vi "PMT_plus_Kiethley.vi"() -> ()   [LabVIEW 2024]
uses:
  <vilib>/Analysis/NI_AALBase.lvlib
  <vilib>/Analysis/1siggen.llb/Ramp Pattern by Delta.vi
  <vilib>/Utility/file.llb/Write Delimited Spreadsheet (string).vi
  <vilib>/Utility/file.llb/Write Delimited Spreadsheet (DBL).vi
  <userlib>/H11890api/H11890api.lvlib
panel:
  in  "Time to wait before current meas (ms)":i32
  in  "Use PMT?":bool=TRUE
  out "XY Graph":cluster{dbl[], dbl[]}(graph)
  out "Actual Voltage":dbl
  in  "Num Current Meas":i32=6
  in  "Path":path
  out "error out":errorcluster
  in  "VISA resource name":refnum<visa-resource-name>
  out "Set Voltage":dbl
  in  "Step Size (V)":dbl=0.1 format="%#_13g"
  in  "Max V":dbl format="%#_13g"
  in  "Start V":dbl format="%#_13g"
  out "current":dbl
  in  "measurement interval":i32=200
  in  "Source Limit Level (0.1)":dbl=5e-08
  out "standard deviation":dbl
  out "mean":dbl
  out "data":u32[](array[numeric])
  out "OLD":bool
  out "DB":u32[](array[numeric])
  out "Overload":i32
  out "Gate Number":i32
  in  "Correction":bool=TRUE
  out "Num Gates Read":i32
  out "Gate Time Read":i32 caption="Gate time Read"
  out "Num Gates Set":i32=20
  out "Gate Time Set":i32=200
  out "PowerD":i32 caption="Power\nRead Data"
  out "Handle Number":i32
  # "as of now it only records every 1V"
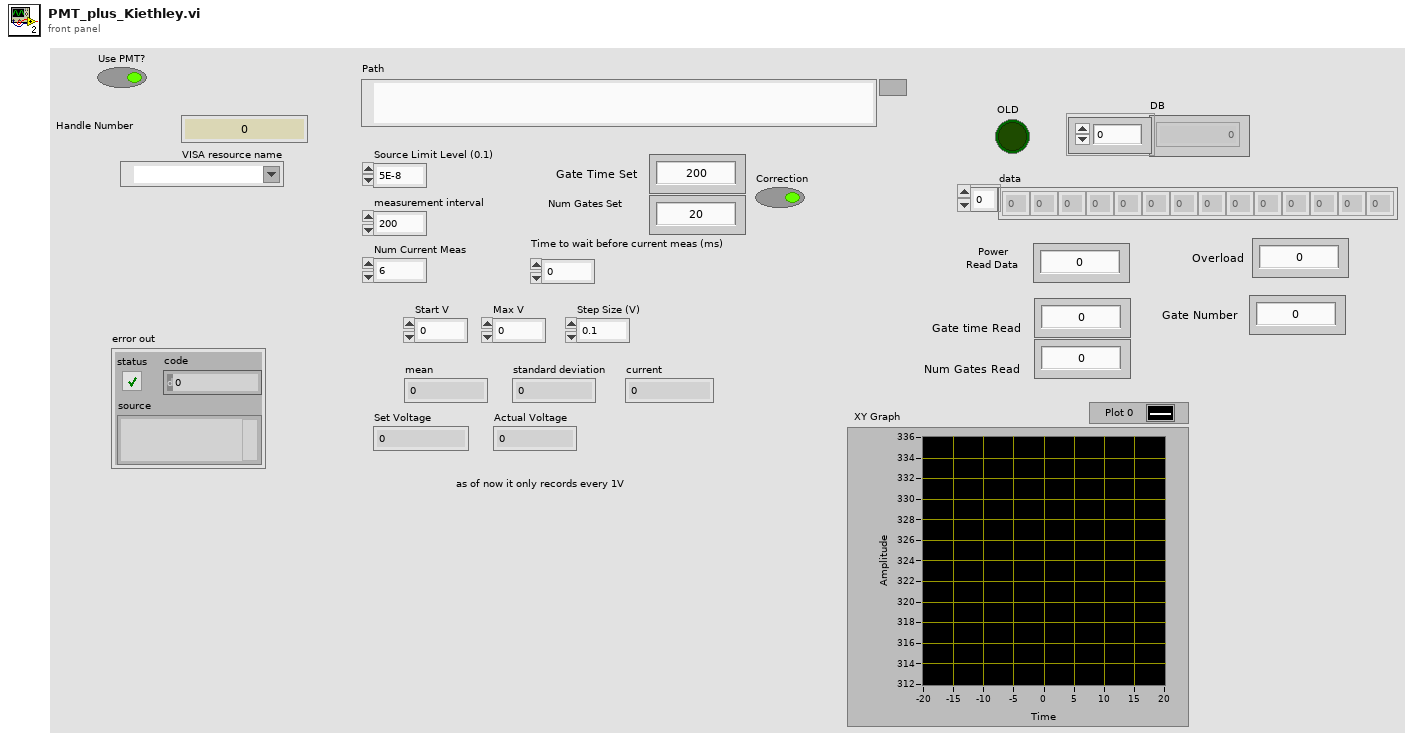
[diagram p1: front panel]
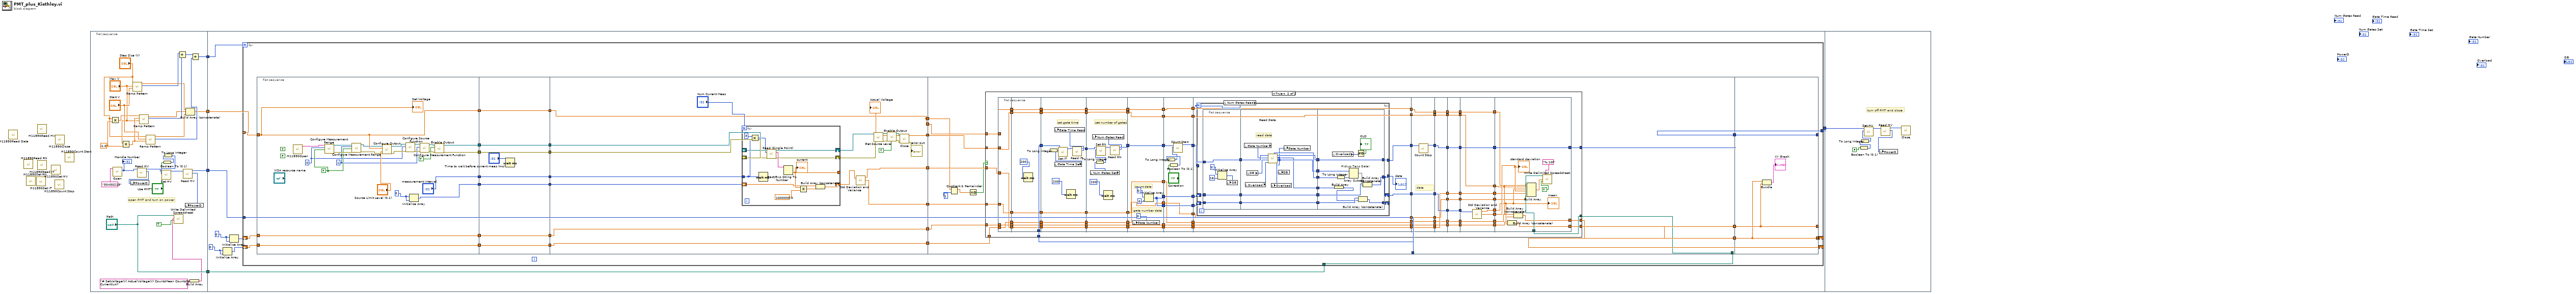
[diagram p0: block diagram]
diagram:
  n1 = call <userlib>:"H11890Read Data.vi"() -> ()  [unwired: 7 in, 5 out]
  n2 = call <userlib>:"H11890Read RN.vi"() -> ()  [unwired: 9 in, 3 out]
  n3 = call <userlib>:"H11890Set RN.vi"() -> ()  [unwired: 10 in, 2 out]
  n4 = call <userlib>:"H11890Set IT.vi"() -> ()  [unwired: 10 in, 2 out]
  n5 = call <userlib>:"H11890Read HV.vi"() -> ()  [unwired: 9 in, 3 out]
  n6 = call <userlib>:"H11890Read IT.vi"() -> ()  [unwired: 9 in, 3 out]
  n7 = call <userlib>:"H11890Set HV.vi"() -> ()  [unwired: 10 in, 2 out]
  n8 = call <userlib>:"H11890Count Stop.vi"() -> ()  [unwired: 10 in, 2 out]
  n9 = call <userlib>:"H11890Close.vi"() -> ()  [unwired: 10 in, 2 out]
  n10 = call <userlib>:"H11890Count Start.vi"() -> ()  [unwired: 10 in, 2 out]
  n11 = flat-sequence {
    tunnel: [w25] -> w5
    tunnel: [w14] -> w4
    tunnel: [w13] -> w3
    tunnel: ["Path"] -> w1
    tunnel: w5 -> [w43]
    tunnel: w4 -> [w42]
    tunnel: w3 -> [w41]
    tunnel: [w40] -> w2
    tunnel: w1 -> [w39]
    tunnel: w2 -> [w434]
    frame #0 {
      w8 = -1.0
      # "open PMT and turn on power"
      n12 = Multiply(x="Step Size (V)", y=w8) -> (x*y=w6:dbl)
      n13 = call "Open.vi"("Serial Number"="30430219") -> ("Handle Number"=w29:i32)  [unwired: 9 in, 1 out]
      "Handle Number" <- w29
      n14 = Multiply(x="Max V", y=w8) -> (x*y=w16:dbl)
      n15 = call-poly <vilib>:"Ramp Pattern.vi"("start"="Start V", "end"="Max V", "delta"="Step Size (V)") -> ("samples"=w21:i32, "Ramp Pattern"=w18:dbl[])  [unwired: 6 in, 1 out]
      n16 = call "Read HV.vi"("handle"=w29) -> ("HV out"=w28:i32, "handle out"=w32:i32)  [unwired: 8 in, 1 out]
      n17 = local write "PowerD"(w28) -> ()
      n18 = call-poly <vilib>:"Ramp Pattern.vi"("start"="Max V", "end"=w16, "delta"=w6) -> ("samples"=w22:i32, "Ramp Pattern"=w19:dbl[])  [unwired: 6 in, 1 out]
      n19 = call-poly <vilib>:"Ramp Pattern.vi"("start"=w16, "end"="Start V", "delta"="Step Size (V)") -> ("samples"=w24:i32, "Ramp Pattern"=w20:dbl[])  [unwired: 6 in, 1 out]
      n20 = Boolean To (0,1)(Boolean="Use PMT?") -> (0, 1=w30:i16)
      n21 = To Long Integer(number=w30) -> (32bit integer=w31:i32)
      n22 = call "Set HV.vi"("HV"=w31, "handle"=w32) -> ("handle out"=w34:i32)  [unwired: 8 in, 1 out]
      n23 = Add(x=w21, y=w22) -> (x+y=w23:i32)
      n24 = call "Read HV.vi"("handle"=w34) -> ("HV out"=w33:i32, "handle out"=w25:i32)  [unwired: 8 in, 1 out]
      n25 = local write "PowerD"(w33) -> ()
      n26 = Build Array (concatenate)(w18, w19, w20) -> (w14:dbl[])
      n27 = Build Array("# SetVoltage(V) ActualVoltage(V) CountsMean CountsStd Current(uA)") -> (w10:string[])
      n28 = call-poly <vilib>:"Write Delimited Spreadsheet.vi"("file path (dialog if empty)"="Path", "1D data"=w10, "append to file? (new file:F)"=TRUE) -> ()  [unwired: 11 in, 2 out]
      n29 = Add(x=w23, y=w24) -> (x+y=w13:i32)
    }
    frame #1 {
      w37 = 0
      w38 = 0
      n30 = Initialize Array(w37, w37) -> (w36:i32[])
      n31 = Initialize Array(w38, w38) -> (w35:i32[])
      n32 = for {
        N: w41 -> [_]
        tunnel: w42 -> [w75] mode=indexing
        tunnel: w43 -> [w74]
        tunnel: [w73] -> w40
        tunnel: w39 -> [w72]
        shift-right: [w59] -> _
        shift-left: w35 -> [w67]
        shift-right: [w60] -> _
        shift-left: w36 -> [w66]
        n33 = flat-sequence {
          tunnel: w66 -> [w99]
          tunnel: w67 -> [w100]
          tunnel: w75 -> [w101]
          tunnel: [w101] -> w58
          tunnel: [w100] -> w56
          tunnel: [w99] -> w54
          tunnel: ["measurement interval"] -> w52
          tunnel: [w79] -> w50
          tunnel: [w78] -> w48
          tunnel: [w77] -> w46
          tunnel: w58 -> [w109]
          tunnel: [w109] -> w57
          tunnel: w56 -> [w108]
          tunnel: [w108] -> w55
          tunnel: w54 -> [w107]
          tunnel: [w107] -> w53
          tunnel: w52 -> [w106]
          tunnel: [w106] -> w51
          tunnel: w50 -> [w105]
          tunnel: [w105] -> w49
          tunnel: w48 -> [w104]
          tunnel: [w104] -> w47
          tunnel: w46 -> [w103]
          tunnel: [w103] -> w45
          tunnel: [w119] -> w71
          tunnel: [w120] -> w70
          tunnel: [w112] -> w69
          tunnel: [w119] -> w68
          tunnel: [w118] -> w65
          tunnel: [w117] -> w64
          tunnel: w57 -> [w119]
          tunnel: w55 -> [w118]
          tunnel: w53 -> [w117]
          tunnel: w51 -> [w116]
          tunnel: w49 -> [w115]
          tunnel: w47 -> [w114]
          tunnel: w45 -> [w113]
          tunnel: [w110] -> w44
          tunnel: w74 -> [w157]
          tunnel: w72 -> [w155]
          tunnel: w71 -> [w154]
          tunnel: w70 -> [w153]
          tunnel: w69 -> [w152]
          tunnel: w68 -> [w149]
          tunnel: w65 -> [w147]
          tunnel: w64 -> [w146]
          tunnel: [w156] -> w63
          tunnel: [w145] -> w62
          tunnel: [w144] -> w61
          tunnel: w44 -> [w143]
          tunnel: [w431] -> w59
          tunnel: [w432] -> w60
          tunnel: [w433] -> w73
          tunnel: w63 -> [w433]
          tunnel: w62 -> [w432]
          tunnel: w61 -> [w431]
          frame #0 {
            w85 = 0
            w84 = TRUE
            w81 = 1
            w83 = 0
            (unwired) FALSE
            (unwired) TRUE
            n34 = call <userlib>:"H11890Open.vi"() -> ("cSerialNumber out"=w76:string)  [unwired: 10 in, 1 out]
            n35 = call "Configure Measurement Range.vi"("Enable Auto Range (T:Enable)"=w84, "Function (0: Volts)"=w83, "VISA resource name"=w76) -> ("error out"=w96:errorcluster, "VISA resource name out"=w95:refnum<visa-resource-name>, "error in (no error)"=w97:errorcluster)  [unwired: 6 in]
            n36 = call "Configure Measurement Range.vi"("error in (no error)"=w96, "Enable Auto Range (T:Enable)"=w84, "Function (0: Volts)"=w81, "VISA resource name"=w95) -> ("error out"=w91:errorcluster, "VISA resource name out"=w87:refnum<visa-resource-name>)  [unwired: 6 in]
            n37 = call "Configure Output.vi"("VISA resource name"=w87, "Source Level (0)"=w101, "Source Limit Level (0.1)"="Source Limit Level (0.1)", "error in (no error)"=w91) -> ("VISA resource name out"=w88:refnum<visa-resource-name>, "error out"=w92:errorcluster)  [unwired: 10 in]
            n38 = call "Configure Source Function.vi"("error in (no error)"=w92, "Function (0: Volts)"=w83, "VISA resource name"=w88) -> ("error out"=w93:errorcluster, "VISA resource name out"=w89:refnum<visa-resource-name>)  [unwired: 7 in]
            n39 = Initialize Array(w85, w85) -> (w79:i32[])
            n40 = call "Configure Measurement Function.vi"("error in (no error)"=w93, "Function (0: Volts)"=w81, "VISA resource name"=w89) -> ("error out"=w94:errorcluster, "VISA resource name out"=w90:refnum<visa-resource-name>)  [unwired: 7 in]
            n41 = call "Enable Output.vi"("error in (no error)"=w94, "Enable Output (T: Enable)"=TRUE, "VISA resource name"=w90) -> ("error out"=w78:errorcluster, "VISA resource name out"=w77:refnum<visa-resource-name>)  [unwired: 7 in]
            "Set Voltage" <- w101
          }
          frame #1 {
            n42 = Wait (ms)(milliseconds to wait="Time to wait before current meas (ms)") -> ()  [unwired: 1 out]
          }
          frame #2 {
            n43 = for {
              N: "Num Current Meas" -> [_]
              tunnel: [w131] -> _
              shift-right: [w141] -> w126
              shift-left: w114 -> [w140]
              shift-right: [w139] -> w129
              shift-left: w113 -> [w138]
              tunnel: w116 -> [w135]
              shift-right: [w133] -> w111
              shift-left: w115 -> [w134]
              n44 = Multiply(x=3, y=w135) -> (x*y=w137:i32)
              n45 = Wait (ms)(milliseconds to wait=w135) -> ()  [unwired: 1 out]
              n46 = call "Read (Single Point).vi"("VISA resource name"=w138, "Timeout (10000 ms)"=w137, "error in (no error)"=w140) -> ("VISA resource name out"=w139:refnum<visa-resource-name>, "Data out"=w142:string, "error out"=w141:errorcluster)  [unwired: 10 in]
              n47 = Fract/Exp String To Number(string=w142) -> (number=w131:dbl)  [unwired: 3 in, 1 out]
              "current" <- w131
              n48 = Multiply(x=w131, y=1000000.0) -> (x*y=w130:dbl)
              n49 = Build Array (concatenate)(w134, w130) -> (w133:dbl[])
            }
            n50 = call <vilib>:"Std Deviation and Variance.vi"("X"=w111) -> ("mean"=w112:dbl, "standard deviation"=w110:dbl)  [unwired: 1 in, 1 out]
            n51 = call "Get Source Level.vi"("error in (no error)"=w126, "VISA resource name"=w129) -> ("error out"=w127:errorcluster, "Voltage Level Out"=w120:dbl, "VISA resource name out"=w128:refnum<visa-resource-name>)  [unwired: 6 in, 1 out]
            "Actual Voltage" <- w120
            n52 = call "Enable Output.vi"("error in (no error)"=w127, "Enable Output (T: Enable)"=TRUE, "VISA resource name"=w128) -> ("error out"=w122:errorcluster, "VISA resource name out"=w123:refnum<visa-resource-name>)  [unwired: 7 in]
            n53 = call "Close.vi"("error in (no error)"=w122, "VISA resource name"=w123) -> ("error out"=→"error out":errorcluster)  [unwired: 9 in]
          }
          frame #3 {
            n54 = Quotient & Remainder(x=w149, y=1) -> (x-y*floor(x/y)=w151:dbl)  [unwired: 1 out]
            n55 = Equal To 0?(x=w151) -> (x = 0?=w150:bool)
            n56 = case shown="True" w150 {
              tunnel: w157 -> [w160 w204]
              tunnel: [w160 w203] -> w156
              tunnel: w155 -> [_ w202]
              tunnel: w154 -> [_ w201]
              tunnel: w153 -> [_ w200]
              tunnel: w152 -> [_ w199]
              tunnel: w147 -> [w159 w198]
              tunnel: w146 -> [w158 w186]
              tunnel: [w159 w174] -> w145
              tunnel: [w158 w173] -> w144
              tunnel: w143 -> [_ w172]
              frame False {
              }
              frame True {
                n57 = flat-sequence {
                  tunnel: [w263] -> w257
                  tunnel: [w261] -> w256
                  tunnel: [w262] -> w255
                  tunnel: w201 -> [w263]
                  tunnel: w200 -> [w262]
                  tunnel: w199 -> [w261]
                  tunnel: w198 -> [w260]
                  tunnel: [w260] -> w187
                  tunnel: w186 -> [w259]
                  tunnel: [w259] -> w179
                  tunnel: w172 -> [w258]
                  tunnel: [w258] -> w168
                  tunnel: [w270] -> w254
                  tunnel: w204 -> [w270]
                  tunnel: [w269] -> w253
                  tunnel: w257 -> [w269]
                  tunnel: [w268] -> w252
                  tunnel: w256 -> [w268]
                  tunnel: [w267] -> w251
                  tunnel: w255 -> [w267]
                  tunnel: [w266] -> w188
                  tunnel: w187 -> [w266]
                  tunnel: [w265] -> w180
                  tunnel: w179 -> [w265]
                  tunnel: [w264] -> w169
                  tunnel: w168 -> [w264]
                  tunnel: w254 -> [w284]
                  tunnel: [w279] -> w250
                  tunnel: [w277] -> w249
                  tunnel: w253 -> [w277]
                  tunnel: [w276] -> w248
                  tunnel: w252 -> [w276]
                  tunnel: [w275] -> w247
                  tunnel: w251 -> [w275]
                  tunnel: [w274] -> w189
                  tunnel: w188 -> [w274]
                  tunnel: [w273] -> w181
                  tunnel: w180 -> [w273]
                  tunnel: [w272] -> w170
                  tunnel: w169 -> [w272]
                  tunnel: [w293] -> w246
                  tunnel: w250 -> [w295]
                  tunnel: [w290] -> w245
                  tunnel: w249 -> [w290]
                  tunnel: w248 -> [w289]
                  tunnel: [w289] -> w244
                  tunnel: [w288] -> w243
                  tunnel: w247 -> [w288]
                  tunnel: [w287] -> w190
                  tunnel: w189 -> [w287]
                  tunnel: [w286] -> w182
                  tunnel: w181 -> [w286]
                  tunnel: [w285] -> w171
                  tunnel: w170 -> [w285]
                  tunnel: w246 -> [w308]
                  tunnel: [w308] -> w242
                  tunnel: [w304] -> w241
                  tunnel: [w304] -> w240
                  tunnel: [w303] -> w239
                  tunnel: w245 -> [w303]
                  tunnel: [w302] -> w238
                  tunnel: w244 -> [w302]
                  tunnel: w243 -> [w301]
                  tunnel: [w301] -> w237
                  tunnel: [w300] -> w191
                  tunnel: w190 -> [w300]
                  tunnel: [w299] -> w183
                  tunnel: w182 -> [w299]
                  tunnel: w171 -> [w298]
                  tunnel: [w298] -> w164
                  tunnel: w242 -> [w321]
                  tunnel: [w317] -> w236
                  tunnel: w241 -> [w316]
                  tunnel: w240 -> [w315]
                  tunnel: [w316] -> w235
                  tunnel: [w315] -> w234
                  tunnel: w239 -> [w314]
                  tunnel: [w314] -> w233
                  tunnel: [w313] -> w232
                  tunnel: w238 -> [w313]
                  tunnel: [w312] -> w231
                  tunnel: w237 -> [w312]
                  tunnel: [w311] -> w192
                  tunnel: w191 -> [w311]
                  tunnel: [w310] -> w184
                  tunnel: w183 -> [w310]
                  tunnel: [w309] -> w165
                  tunnel: w164 -> [w309]
                  tunnel: [w334] -> w230
                  tunnel: w236 -> [w333]
                  tunnel: w235 -> [w332]
                  tunnel: w234 -> [w331]
                  tunnel: [w330] -> w229
                  tunnel: [w327] -> w228
                  tunnel: w233 -> [w327]
                  tunnel: [w326] -> w227
                  tunnel: w232 -> [w326]
                  tunnel: w231 -> [w325]
                  tunnel: [w325] -> w226
                  tunnel: [w324] -> w193
                  tunnel: w192 -> [w324]
                  tunnel: [w323] -> w185
                  tunnel: w184 -> [w323]
                  tunnel: [w322] -> w166
                  tunnel: w165 -> [w322]
                  tunnel: w230 -> [w388]
                  tunnel: [w387] -> w225
                  tunnel: [w386] -> w224
                  tunnel: w229 -> [w386]
                  tunnel: w228 -> [w385]
                  tunnel: [w385] -> w223
                  tunnel: [w384] -> w222
                  tunnel: w227 -> [w384]
                  tunnel: [w383] -> w221
                  tunnel: w226 -> [w383]
                  tunnel: [w382] -> w194
                  tunnel: w193 -> [w382]
                  tunnel: w185 -> [w381]
                  tunnel: [w381] -> w176
                  tunnel: [w380] -> w167
                  tunnel: w166 -> [w380]
                  tunnel: w225 -> [w395]
                  tunnel: w224 -> [w396]
                  tunnel: [w396] -> w220
                  tunnel: [w395] -> w219
                  tunnel: [w394] -> w218
                  tunnel: w223 -> [w394]
                  tunnel: w222 -> [w393]
                  tunnel: [w393] -> w217
                  tunnel: w221 -> [w392]
                  tunnel: [w392] -> w216
                  tunnel: [w391] -> w195
                  tunnel: w194 -> [w391]
                  tunnel: [w390] -> w177
                  tunnel: w176 -> [w390]
                  tunnel: w167 -> [w389]
                  tunnel: [w389] -> w161
                  tunnel: [w404] -> w215
                  tunnel: w220 -> [w404]
                  tunnel: [w403] -> w214
                  tunnel: w219 -> [w403]
                  tunnel: [w402] -> w213
                  tunnel: w218 -> [w402]
                  tunnel: [w401] -> w212
                  tunnel: w217 -> [w401]
                  tunnel: [w400] -> w211
                  tunnel: w216 -> [w400]
                  tunnel: [w399] -> w196
                  tunnel: w195 -> [w399]
                  tunnel: [w398] -> w178
                  tunnel: w177 -> [w398]
                  tunnel: [w397] -> w162
                  tunnel: w161 -> [w397]
                  tunnel: w215 -> [w414]
                  tunnel: [w413] -> w210
                  tunnel: [w412] -> w209
                  tunnel: [w411] -> w208
                  tunnel: w214 -> [w411]
                  tunnel: [w410] -> w207
                  tunnel: w213 -> [w410]
                  tunnel: [w409] -> w206
                  tunnel: w212 -> [w409]
                  tunnel: [w408] -> w205
                  tunnel: w211 -> [w408]
                  tunnel: [w407] -> w197
                  tunnel: w196 -> [w407]
                  tunnel: w178 -> [w406]
                  tunnel: [w406] -> w175
                  tunnel: [w405] -> w163
                  tunnel: w162 -> [w405]
                  tunnel: w210 -> [w419]
                  tunnel: w209 -> [w427]
                  tunnel: [w429] -> w203
                  tunnel: w208 -> [w429]
                  tunnel: w202 -> [w428]
                  tunnel: w207 -> [w422]
                  tunnel: w206 -> [w425]
                  tunnel: w205 -> [w418]
                  tunnel: w197 -> [w421]
                  tunnel: w175 -> [w420]
                  tunnel: [w417] -> w174
                  tunnel: [w416] -> w173
                  tunnel: w163 -> [w415]
                  frame #0 {
                  }
                  frame #1 {
                    n58 = Wait (ms)(milliseconds to wait=u32 200) -> ()  [unwired: 1 out]
                  }
                  frame #2 {
                    # "set gate time"
                    n59 = local read "Gate Time Set"() -> (w281:i32)
                    n60 = To Long Integer(number=w281) -> (32bit integer=w282:i32)
                    n61 = call "Set IT.vi"("IT"=w282, "handle"=w284) -> ("handle out"=w283:i32)  [unwired: 8 in, 1 out]
                    n62 = Wait (ms)(milliseconds to wait=u32 200) -> ()  [unwired: 1 out]
                    n63 = call "Read IT.vi"("handle"=w283) -> ("IT out"=w280:i32, "handle out"=w279:i32)  [unwired: 8 in, 1 out]
                    n64 = local write "Gate Time Read"(w280) -> ()
                  }
                  frame #3 {
                    # "set number of gates"
                    n65 = local read "Num Gates Set"() -> (w297:i32)
                    n66 = To Long Integer(number=w297) -> (32bit integer=w296:i32)
                    n67 = call "Set RN.vi"("RN"=w296, "handle"=w295) -> ("handle out"=w294:i32)  [unwired: 8 in, 1 out]
                    n68 = Wait (ms)(milliseconds to wait=u32 200) -> ()  [unwired: 1 out]
                    n69 = call "Read RN.vi"("handle"=w294) -> ("RN out"=w292:i32, "handle out"=w293:i32)  [unwired: 8 in, 1 out]
                    n70 = local write "Num Gates Read"(w292) -> ()
                  }
                  frame #4 {
                    # "gate number data"
                    # "count data"
                    n71 = local write "Gate Number"(0) -> ()
                    n72 = Initialize Array(u32 0, 0 ("次元サイズ")) -> (w304:u32[])
                  }
                  frame #5 {
                    n73 = Boolean To (0,1)(Boolean="Correction") -> (0, 1=w320:i16)
                    n74 = To Long Integer(number=w320) -> (32bit integer=w319:i32)
                    n75 = call "Count Start.vi"("Correction"=w319, "handle"=w321) -> ("handle out"=w317:i32)  [unwired: 8 in, 1 out]
                  }
                  frame #6 {
                    n76 = local read "Num Gates Read"() -> (w329:i32)
                    n77 = for {
                      N: w329 -> [_]
                      shift-right: [w335] -> w330
                      shift-left: w332 -> [w343]
                      shift-right: [w339] -> _
                      shift-left: w331 -> [w342]
                      tunnel: w333 -> [w344]
                      tunnel: [w345] -> w334
                      tunnel: [w335] -> w328
                      n78 = flat-sequence {
                        tunnel: [w355] -> w349
                        tunnel: [w354] -> w340
                        tunnel: [w353] -> w337
                        tunnel: w344 -> [w355]
                        tunnel: w343 -> [w354]
                        tunnel: w342 -> [w353]
                        tunnel: [w366] -> w348
                        tunnel: w349 -> [w365]
                        tunnel: [w360] -> w347
                        tunnel: [w359] -> w346
                        tunnel: [w358] -> w341
                        tunnel: w340 -> [w358]
                        tunnel: [w357] -> w338
                        tunnel: w337 -> [w357]
                        tunnel: [w356] -> w336
                        tunnel: w348 -> [w379]
                        tunnel: w347 -> [w374]
                        tunnel: w346 -> [w373]
                        tunnel: w341 -> [w371]
                        tunnel: w338 -> [w370]
                        tunnel: w336 -> [w369]
                        tunnel: [w379] -> w345
                        tunnel: [w372] -> w335
                        tunnel: [w367] -> w339
                        frame #0 {
                          n79 = Initialize Array(u32 0, 16 ("次元サイズ")) -> (w350:u32[])
                          n80 = local write "DB"(w350) -> ()
                        }
                        frame #1 {
                          # "read data"
                          n81 = local read "Gate Number"() -> (w364:i32)
                          n82 = local read "Overload"() -> (w363:i32)
                          n83 = local read "DB"() -> (w361:u32[])
                          n84 = call "Read Data.vi"("OLD"=w363, "DataBuf"=w361, "GateNum"=w364, "handle"=w365) -> ("OLD out"=w362:i32, "DataBuf out"=w359:u32[], "GateNum out"=w356:i32, "handle out"=w366:i32, "function return"=w360:u32)  [unwired: 3 in]
                          n85 = local write "Overload"(w362) -> ()
                          n86 = local write "DB"(w359) -> ()
                          n87 = local write "Gate Number"(w356) -> ()
                        }
                        frame #2 {
                          # "Pickup Tans Data!"
                          n88 = local read "Overload"() -> (w377:i32)
                          n89 = Build Array(w369) -> (w368:i32[])
                          n90 = To Long Integer(number=w374) -> (32bit integer=w375:i32)
                          n91 = Array Subset(array=w373, length=w375) -> (w376:u32[])  [unwired: 1 in]
                          n92 = Not Equal To 0?(x=w377) -> (x != 0?=→"OLD":bool)
                          n93 = Build Array (concatenate)(w370, w368) -> (w367:u32[])
                          n94 = Build Array (concatenate)(w371, w376) -> (w372:u32[])
                        }
                      }
                    }
                    "data" <- w328
                  }
                  frame #7 {
                    # "data"
                    n95 = call "Count Stop.vi"("handle"=w388) -> ("handle out"=w387:i32)  [unwired: 9 in, 1 out]
                  }
                  frame #8 {
                  }
                  frame #9 {
                  }
                  frame #10 {
                    n96 = call <vilib>:"Std Deviation and Variance.vi"("X"=w414) -> ("mean"=w413:dbl, "standard deviation"=w412:dbl)  [unwired: 1 in, 1 out]
                  }
                  frame #11 {
                    n97 = Build Array (concatenate)(w421, w419) -> (w416:dbl[])
                    n98 = Build Array (concatenate)(w420, w418) -> (w417:dbl[])
                    n99 = Build Array(w422, w418, w419, w427, w425, w415) -> (w426:dbl[])
                    n100 = call-poly <vilib>:"Write Delimited Spreadsheet.vi"("file path (dialog if empty)"=w428, "format (%.3f)"="%.10f", "1D data"=w426, "append to file? (new file:F)"=TRUE) -> ()  [unwired: 10 in, 2 out]
                    "mean" <- w419
                    "standard deviation" <- w427
                  }
                }
              }
            }
          }
          frame #4 {
            n101 = Bundle(w432, w431) -> (→"XY Graph":cluster{dbl[], dbl[]})  [unwired: 1 in]
          }
        }
      }
    }
    frame #2 {
      # "turn off PMT and close"
      n102 = Boolean To (0,1)(Boolean=FALSE) -> (0, 1=w439:i16)
      n103 = To Long Integer(number=w439) -> (32bit integer=w438:i32)
      n104 = call "Set HV.vi"("HV"=w438, "handle"=w434) -> ("handle out"=w436:i32)  [unwired: 8 in, 1 out]
      n105 = call "Read HV.vi"("handle"=w436) -> ("HV out"=w440:i32, "handle out"=w435:i32)  [unwired: 8 in, 1 out]
      n106 = local write "PowerD"(w440) -> ()
      n107 = call "Close.vi"("Handle"=w435) -> ()  [unwired: 9 in, 2 out]
    }
  }
